vi "readDataArray.vi"(8 "error in (no error)":errorcluster, 10 "array":string[][](array[string]), 11 "DDSFileReader in":refnum<class "DDSFileReader.lvclass">) -> (0 "error out":errorcluster, 3 "DDSFileReader out":refnum<class "DDSFileReader.lvclass">)   [LabVIEW 2011, in "Tools.lvlib" / "Filing.lvlib" / "DDSFileReader.lvclass"]
uses:
  DDSFileReader.lvclass
  Hal/Channels/DDSOutput/Generic/DDSOutput.lvclass
  DDSFileReader.lvclass/DDSFileReader.ctl
panel:
  out "Defaults":T1(array[cluster])
  out "Data":T2(array[cluster])
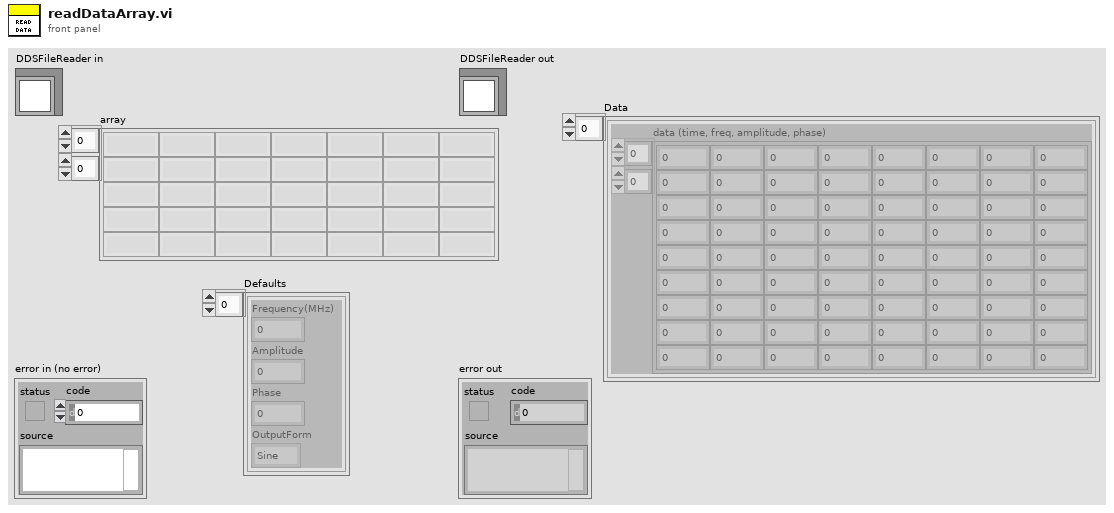
[diagram p1: front panel]
types:
  T1 = cluster{"Frequency(MHz)":dbl, "Amplitude":dbl, "Phase":dbl, "OutputForm":enum16{"Sine", "Square", "Triangle", "Arbitrary"}}[]
  T2 = cluster{"data (time, freq, amplitude, phase)":dbl[][]}[]
  T3 = cluster{"OutputForm":enum16{"Sine", "Square", "Triangle", "Arbitrary"}[], "OutputFunction":enum16{"Frequency", "Ramp", "Sequence"}[], "physicalChannels":string}
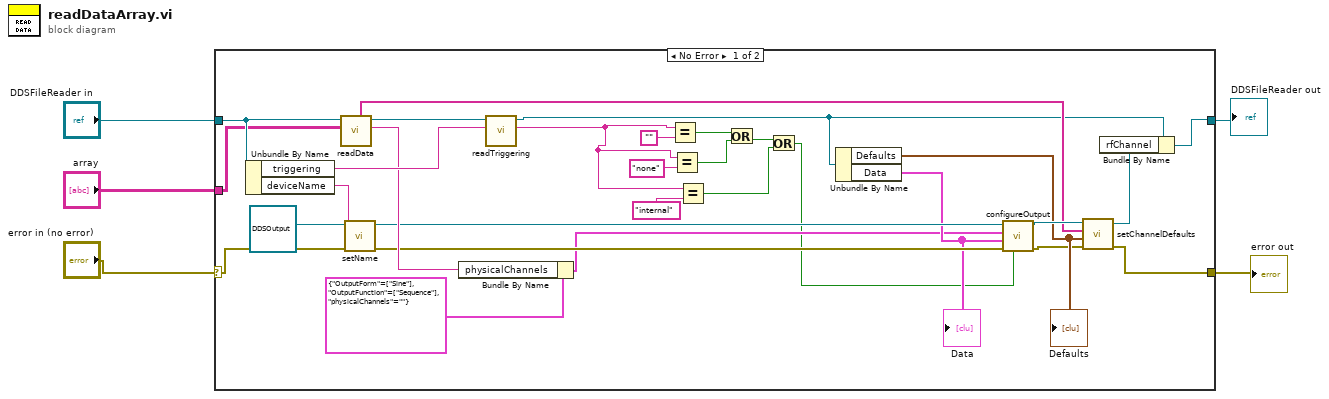
[diagram p0: block diagram]
diagram:
  n1 = case shown="No Error" "error in (no error)" {
    selector: "error in (no error)" -> [w19 w36]
    tunnel: "array" -> [w17 _]
    tunnel: "DDSFileReader in" -> [w25 w37]
    tunnel: [w6 w37] -> w2
    tunnel: [w9 w36] -> w1
    frame No Error {
      n2 = Unbundle By Name(w25) -> ("triggering"=w24:string, "deviceName"=w23:string)
      n3 = call-dynamic "readData.vi"("array"=w17, "DDSFileReader in"=w25) -> ("channels"=w21:string, "DDSFileReader out"=w26:refnum<class "DDSFileReader.lvclass">, "channelAddresses"=w11:string[])  [unwired: 4 in, 3 out]
      n4 = call "setName.vi"("error in (no error)"=w19, "name"=w23, "DDSOutput in"=refnum<class "DDSOutput.lvclass"> refnum) -> ("error out"=w18:errorcluster, "DDSOutput out"=w20:refnum<class "DDSOutput.lvclass">)  [unwired: 7 in]
      n5 = Bundle By Name(cluster=T3 {"OutputForm"=[enum."Sine"], "OutputFunction"=[enum."Sequence"], "physicalChannels"=""} ("Config"), "physicalChannels"=w21) -> (w15:T3)
      n6 = call-dynamic "readTriggering.vi"("triggering"=w24, "FileReader in"=w26) -> ("clock source"=w22:string, "FileReader out"=w7:refnum<class "DDSFileReader.lvclass">)  [unwired: 6 in, 2 out]
      n7 = Equal?(x=w22, y="") -> (x = y?=w31:bool)
      n8 = Equal?(x=w22, y="none") -> (x = y?=w30:bool)
      n9 = Equal?(x=w22, y="internal") -> (x = y?=w27:bool)
      n10 = Or(x=w31, y=w30) -> (x .or. y?=w29:bool)
      n11 = Or(x=w29, y=w27) -> (x .or. y?=w14:bool)
      n12 = Unbundle By Name(w7) -> ("Defaults"=w12:T1, "Data"=w16:T2)
      "Data" <- w16
      "Defaults" <- w12
      n13 = call-dynamic "configureOutput.vi"("sofwareTrigger?"=w14, "error in (no error)"=w18, "Data"=w16, "Config"=w15, "DDSOutput in"=w20) -> ("error out"=w10:errorcluster, "DDSOutput out"=w13:refnum<class "DDSOutput.lvclass">)  [unwired: 5 in]
      n14 = call-dynamic "setChannelDefaults.vi"("error in (no error)"=w10, "Data"=w12, "physicalChannels"=w11, "DDSOutput in"=w13) -> ("error out"=w9:errorcluster, "DDSOutput out"=w8:refnum<class "DDSOutput.lvclass">)  [unwired: 6 in]
      n15 = Bundle By Name(cluster=w7, "rfChannel"=w8) -> (w6:refnum<class "DDSFileReader.lvclass">)
    }
    frame Error {
    }
  }
  "error out" <- w1
  "DDSFileReader out" <- w2
